vi "Navigation.vi"(8 "error in (no error)":errorcluster, 9 "Thread 1 Ref":refnum<vi>, 10 "Thread 0 Ref":refnum<vi>, 11 "MyApp in":refnum<class "MyApp.lvclass">) -> (0 "error out":errorcluster, 3 "MyApp out":refnum<class "MyApp.lvclass">)   [LabVIEW 2012, in "MyApp.lvlib" / "MyApp.lvclass"]
uses:
  MyApp.lvclass
  HGF_LVC/HGF_BaseClasses/HGF_Event/HGF_Event.lvclass
  HGF_LVC/HGF_BaseClasses/HGF_Stop/HGF_Stop.lvclass
  <vilib>/Utility/error.llb/DialogType.ctl
  HGF_LVC/HGF_ApplicationBaseClasses/HGF_Application/HGF_Application.lvclass
panel:
  in  "Thread 1":bool
  in  "Top":bool
  out "Iteration":i32
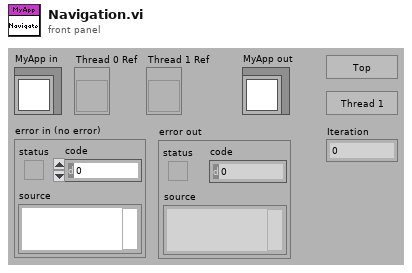
[diagram p1: front panel]
types:
  T1 = cluster{"seconds since 1Jan1904":timestamp, "message":string}
  T2 = typedef "DialogType.ctl" = u16
  T3 = cluster{"seconds since 1Jan1904":timestamp, string}
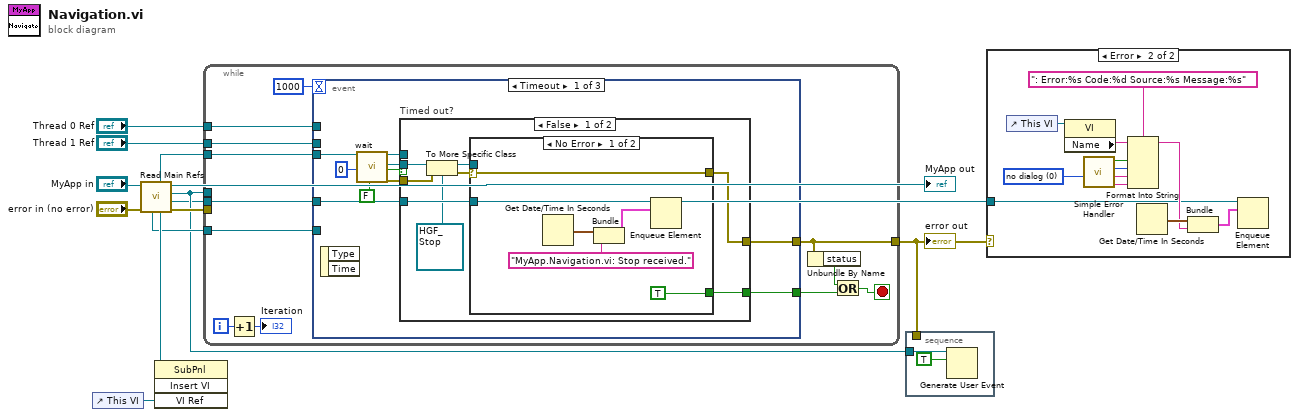
[diagram p0: block diagram]
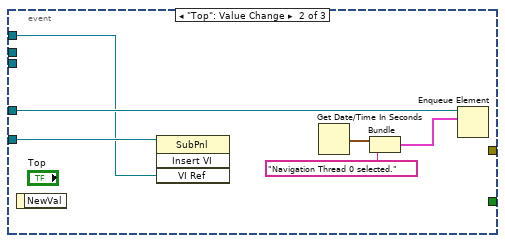
[diagram p5: hidden frame]
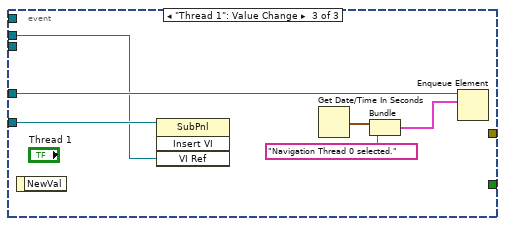
[diagram p6: hidden frame]
diagram:
  n1 = control-ref of="This VI"() -> (w11:refnum<vi>)
  n2 = call "Read Main Refs.vi"("error in (no error)"="error in (no error)", "HGF_Application in"="MyApp in") -> ("error out"=w12:errorcluster, "Status Info Queue"=w2:refnum<queue>, "Main Stop Event"=w3:refnum<user-event>, "HGF_Application out"=→"MyApp out":refnum<class "MyApp.lvclass">, "Navigation Sub Panel"=w7:refnum<vi>, "Info Event"=w13:refnum<class "HGF_Event.lvclass">, "Application Sub Panel"=w6:refnum<vi>)  [unwired: 2 in, 1 out]
  n3 = invoke class="SubPnl" method="Insert VI"(reference=w7, "VI Ref"=w11) -> ()  [unwired: 2 in, 4 out]
  n4 = while {
    tunnel: w3 -> [_]
    tunnel: w13 -> [w23]
    tunnel: w12 -> [_]
    tunnel: w2 -> [w20]
    tunnel: [w16] -> w1
    tunnel: w6 -> [w21]
    tunnel: "Thread 1 Ref" -> [w19]
    tunnel: "Thread 0 Ref" -> [w18]
    i -> [w25]
    stop <- w15 stop-if-true
    n5 = Increment(x=w25) -> (x+1=→"Iteration":i32)
    n6 = event shown="[0] Timeout" {
      selector: _ -> [_ _ _]
      dyn-events: _ -> [_ _ _]
      timeout: 1000 -> [_ _ _]
      tunnel: w23 -> [w31 _ _]
      tunnel: [w30 _ _] -> w16
      tunnel: w21 -> [_ w54 w60]
      tunnel: w20 -> [w27 w53 w59]
      tunnel: w19 -> [_ _ w58]
      tunnel: w18 -> [_ w52 _]
      tunnel: [w28 _ _] -> w17
      event Timeout {
        n7 = event-data() -> ()  [unwired: 1 in, 2 out]
        n8 = call-dynamic "wait.vi"("HGF_Event"=w31, "msTimeout (-1)"=0, "ignore previous (F)"=FALSE) -> ("dup HGF_Event"=w34:refnum<class "HGF_Event.lvclass">, "Object"=w33:refnum<class>, "timed out"=w32:bool, "error out"=w35:errorcluster)  [unwired: 13 in]
        n9 = case "Timed out?" shown="False" w32 {
          tunnel: [w38 w51] -> w30
          tunnel: w35 -> [w42 w51]
          tunnel: w34 -> [_ _]
          tunnel: w33 -> [w43 _]
          tunnel: [w39 _] -> w28
          tunnel: w27 -> [w36 _]
          frame False {
            n10 = To More Specific Class(target class=refnum<class "HGF_Stop.lvclass"> refnum ("HGF_BaseClasses.lvlib:HGF_Stop.lvclass"), reference=w43, error in=w42) -> (specific class reference=w40:refnum<class "HGF_Stop.lvclass">, error out=w41:errorcluster)
            n11 = case shown="No Error" w41 {
              selector: w41 -> [w48 w50]
              tunnel: w40 -> [_ _]
              tunnel: [TRUE _] -> w39
              tunnel: [w48 w50] -> w38
              tunnel: w36 -> [w44 _]
              frame No Error {
                n12 = Get Date/Time In Seconds() -> (seconds since 1Jan1904=w46:timestamp)
                n13 = Bundle("seconds since 1Jan1904"=w46, "message"="MyApp.Navigation.vi: Stop received.") -> (w47:T1)  [unwired: 1 in]
                n14 = Enqueue Element(queue=w44, element=w47) -> ()  [unwired: 2 in, 3 out]
              }
              frame Error {
              }
            }
          }
          frame True {
          }
        }
      }
      event "Top": Value Change {
        n15 = event-data() -> ()  [unwired: 1 in, 1 out]
        n16 = invoke class="SubPnl" method="Insert VI"(reference=w54, "VI Ref"=w52) -> ()  [unwired: 2 in, 4 out]
        n17 = Get Date/Time In Seconds() -> (seconds since 1Jan1904=w57:timestamp)
        n18 = Bundle("seconds since 1Jan1904"=w57, "message"="Navigation Thread 0 selected.") -> (w55:T1)  [unwired: 1 in]
        n19 = Enqueue Element(queue=w53, element=w55) -> ()  [unwired: 2 in, 3 out]
      }
      event "Thread 1": Value Change {
        n20 = event-data() -> ()  [unwired: 1 in, 1 out]
        n21 = invoke class="SubPnl" method="Insert VI"(reference=w60, "VI Ref"=w58) -> ()  [unwired: 2 in, 4 out]
        n22 = Get Date/Time In Seconds() -> (seconds since 1Jan1904=w63:timestamp)
        n23 = Bundle("seconds since 1Jan1904"=w63, "message"="Navigation Thread 0 selected.") -> (w61:T1)  [unwired: 1 in]
        n24 = Enqueue Element(queue=w59, element=w61) -> ()  [unwired: 2 in, 3 out]
      }
    }
    n25 = Unbundle By Name(w16) -> ("status"=w14:bool)
    n26 = Or(x=w14, y=w17) -> (x .or. y?=w15:bool)
  }
  "error out" <- w1
  n27 = stacked-sequence {
    tunnel: w3 -> [w65]
    tunnel: w1 -> [_]
    frame #0 {
      n28 = Generate User Event(user event=w65, event data cluster=TRUE ("event data")) -> ()  [unwired: 1 in, 2 out]
    }
  }
  n29 = case shown="Error" w1 {
    tunnel: w2 -> [_ w66]
    frame No Error {
    }
    frame Error {
      w68 = T2 0 items=["no dialog", "OK message", "continue or stop message", "OK message + warnings", "continue/stop + warnings"] ("type of dialog (OK msg:1)")
      n30 = control-ref of="This VI"() -> (w67:refnum<vi>)
      n31 = property class="VI"(reference=w67) -> ("Name"=w75:string)  [unwired: 1 in, 2 out]
      n32 = call <vilib>:"Simple Error Handler.vi"("type of dialog (OK msg:1)"=w68) -> ("error?"=w74:bool, "code out"=w73:i32, "source out"=w72:string, "message"=w71:string)  [unwired: 4 in, 1 out]
      n33 = Format Into String(format string=": Error:%s Code:%d Source:%s Message:%s", initial string=w75, w74, w73, w72, w71) -> (resulting string=w69:string)  [unwired: 1 in, 1 out]
      n34 = Get Date/Time In Seconds() -> (seconds since 1Jan1904=w77:timestamp)
      n35 = Bundle("seconds since 1Jan1904"=w77, w69) -> (w76:T3)  [unwired: 1 in]
      n36 = Enqueue Element(queue=w66, element=w76) -> ()  [unwired: 2 in, 3 out]
    }
  }
